vi "CANTest2.vi"() -> ()   [LabVIEW 2009, in "Test.lvlib"]
uses:
  Test.lvlib
  <vilib>/Platform/TimedLoop/XDataNode/XDataNode.xnode
  <vilib>/Platform/TimedLoop/XDataNode/loadlvalarms.vi
  <vilib>/Platform/TimedLoop/XDataNode/timing_clust.ctl
  <vilib>/Platform/TimedLoop/XDataNode/nitl_modes.ctl
  <vilib>/Platform/TimedLoop/XDataNode/wakeup.ctl
  <vilib>/Platform/TimedLoop/XDataNode/XDNodeRunTimeDep.lvlib
  CAN.lvlib
  Serial.lvlib
  CAN/SubVIs/CAN Jaguar Control Mode.ctl
panel:
  out "read buffer":u8[](array[numeric])
  out "is Timeout":bool
  out "is Corrupted":bool
  out "read data":u8[](array[numeric]) format="%.0x"
  in  "data":u8[](array[numeric]) format="%.0x"
  in  "messageID":u32 format="%.0x"
  out "error out":errorcluster
  in  "OK Button":bool
  in  "stop 2":bool
  in  "stop":bool
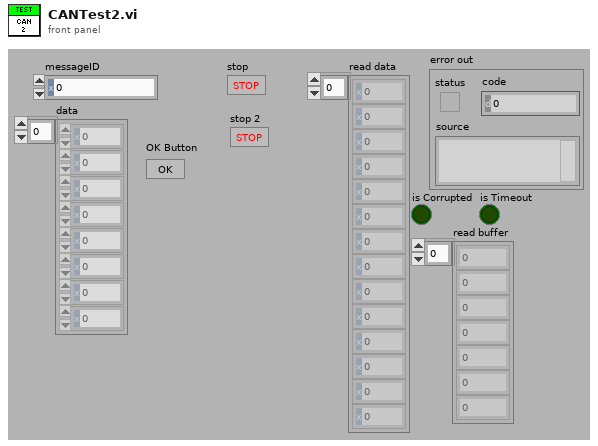
[diagram p1: front panel]
types:
  T1 = typedef "XDNodeRunTimeDep.lvlib/timing_clust.ctl" = cluster{"Expected End [f-1]":u64, "Actual End [f-1]":u64, "Finished Late? [f-1]":bool, "Expected End [i-1]":u64, "Actual End [i-1]":u64, "Finished Late? [i-1]":bool, "Expected Start [i]":u64, "Actual Start [i]":u64, "Expected Start [f]":u64, "Actual Start [f]":u64, "Source Name":string, "Structure Name":string, "Period":i64, "Deadline":i64, "Offset":i64, "Start":i64, "Priority":i32, "Timeout":i32, "Mode":T2, "Wakeup Reason":T3, "Error":errorcluster, "Source Type":string, "Secondary Source Type":string, "Global End Time":u64, "Global Start Time":u64, "Frame Duration":u64, "Iteration Duration":u64, "Assigned CPU":i32, "I/O Scan Engine Mode":u32}
  T2 = typedef "XDNodeRunTimeDep.lvlib/nitl_modes.ctl" = enum32{"No Change", "Process missed periods, maintain original phase", "Discard missed periods, maintain original phase", "Process missed periods, ignore original phase", "Discard missed periods, ignore original phase"}
  T3 = typedef "XDNodeRunTimeDep.lvlib/wakeup.ctl" = enum32{"Normal", "Aborted", "Asynchronous wakeup", "Timing source error", "Timed loop error", "Timeout"}
  T4 = typedef "CAN.lvlib/CAN Jaguar Control Mode.ctl" = enum16{"Percent VBus", "Speed", "Position", "Current"}
  T5 = typedef "CAN.lvlib/CAN Jaguar Ref.ctl" = cluster{"Device Number":u8, "Control Mode":T4, "Inverted":bool, "Semaphore":T6, "Max Vout":dbl, "DevStatus":errorcluster}
  T6 = typedef "Semaphore RefNum" = refnum<k1>
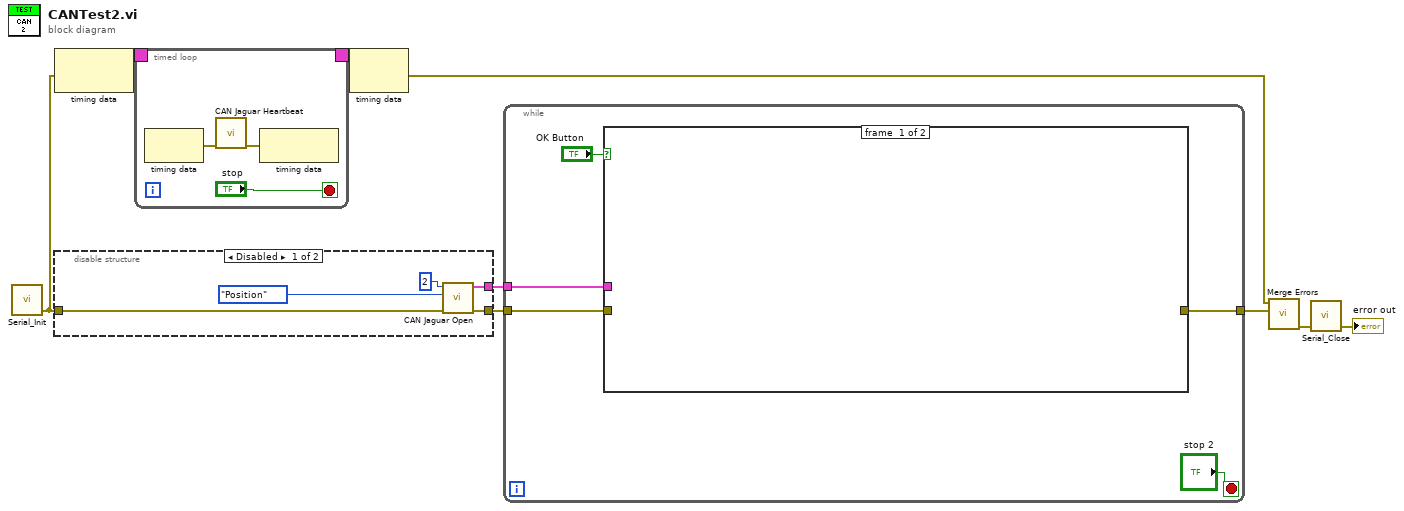
[diagram p0: block diagram]
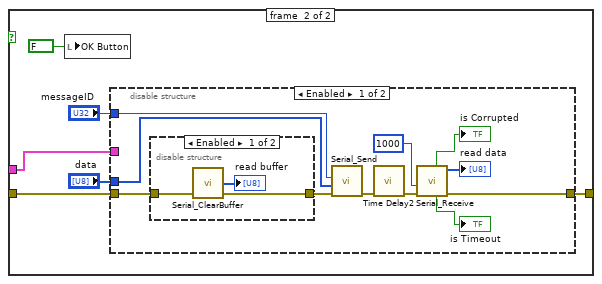
[diagram p3: hidden frame]
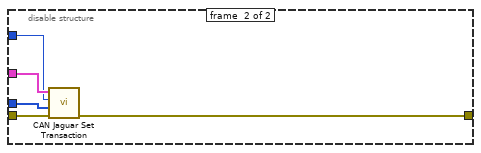
[diagram p5: hidden frame]
diagram:
  n1 = call "Serial_Init.vi"() -> ("error out"=w3:errorcluster)  [unwired: 4 in, 1 out]
  n2 = node-c288(w3) -> (w9:T1)
  n3 = disable-structure shown="Disabled" {
    disable-tunnel: w3 -> [w12 _]
    disable-tunnel: [w11 _] -> w2
    disable-tunnel: [w10 _] -> w1
    frame #0 {
      n4 = call "CAN Jaguar Open.vi"("error in (no error)"=w12, "Control Mode"=CAN_Jaguar_Control_Mode."Position", "Device Number"=u8 2) -> ("error out"=w11:errorcluster, "CAN Jaguar Ref Out"=w10:T5)  [unwired: 7 in]
    }
    frame #1 {
    }
  }
  n5 = timed-loop {
    timing: w9 -> [_]
    timing-out: [_] -> w8
    stop <- "stop" stop-if-true
    n6 = node-c288() -> (w17:errorcluster)  [unwired: 1 in]
    n7 = call "CAN Jaguar Heartbeat.vi"("error in (no error)"=w17) -> ("error out"=w16:errorcluster)  [unwired: 10 in]
    n8 = node-c288(w16) -> ()  [unwired: 1 out]
  }
  n9 = node-c288(w8) -> (w6:errorcluster)
  n10 = while {
    tunnel: [w26] -> w7
    tunnel: w2 -> [w24]
    tunnel: w1 -> [w23]
    stop <- "stop 2" stop-if-true
    n11 = case shown="True" "OK Button" {
      tunnel: [_ w31] -> w26
      tunnel: w24 -> [_ w29]
      tunnel: w23 -> [_ w28]
      frame #0 {
      }
      frame #1 {
        n12 = local write "OK Button"(FALSE ("OK Button")) -> ()
        n13 = disable-structure shown="Enabled" {
          disable-tunnel: "messageID" -> [w44 w50]
          disable-tunnel: "data" -> [w43 w49]
          disable-tunnel: [w42 w52] -> w31
          disable-tunnel: w29 -> [w38 w53]
          disable-tunnel: w28 -> [_ w51]
          frame #0 {
            n14 = disable-structure shown="Enabled" {
              disable-tunnel: w38 -> [w47 w48]
              disable-tunnel: [w45 w48] -> w37
              frame #0 {
                n15 = call "Serial_ClearBuffer.vi"("error in (no error)"=w47) -> ("error out"=w45:errorcluster, "read data"=→"read buffer":u8[])  [unwired: 3 in]
              }
              frame #1 {
              }
            }
            n16 = call "Serial_Send.vi"("error in"=w37, "data"=w43, "messageID"=w44) -> ("error out"=w35:errorcluster)  [unwired: 7 in, 1 out]
            n17 = call "Time Delay2"("error in (no error)"=w35) -> ("error out"=w34:errorcluster)  [unwired: 10 in]
            n18 = call "Serial_Receive.vi"("error in (no error)"=w34, "timeoutMs"=u32 1000) -> ("error out"=w42:errorcluster, "read data"=→"read data":u8[], "is Timeout"=→"is Timeout":bool, "is Corrupted"=→"is Corrupted":bool)  [unwired: 4 in, 2 out]
          }
          frame #1 {
            n19 = call "CAN Jaguar Set Transaction.vi"("error in"=w53, "Data"=w49, "Message ID"=w50, "CAN Jaguar Ref"=w51) -> ("error out"=w52:errorcluster)  [unwired: 6 in, 1 out]
          }
        }
      }
    }
  }
  n20 = call <vilib>:"Merge Errors.vi"("error in 2 (no error)"=w7, "error in 1 (no error)"=w6) -> ("error out"=w4:errorcluster)  [unwired: 5 in]
  n21 = call "Serial_Close.vi"("error in (no error)"=w4) -> ("error out"=→"error out":errorcluster)  [unwired: 4 in]
